vi "_Read Lens Property Settings.vi"() -> (1 "Switches":T1, 2 "Unit":bool, 3 "Spectrum File Path:":path)   [LabVIEW 2015]
uses:
  Type/_Opion Switches.ctl
  <vilib>/Utility/config.llb/Read Key (Path).vi
  <vilib>/Utility/config.llb/Read Key (Boolean).vi
  <vilib>/Utility/config.llb/NI_LVConfig.lvlib
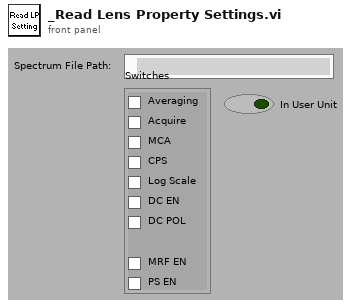
[diagram p1: front panel]
types:
  T1 = typedef "_Opion Switches.ctl" = cluster{"Averaging":bool, "Acquire":bool, "MCA":bool, "CPS":bool, "Log Scale":bool, "DC EN":bool, "DC POL":bool, "MRF EN":bool, "PS EN":bool}
  T2 = typedef "NI_LVConfig.lvlib/Config Data RefNum.ctl" = refnum<k1>
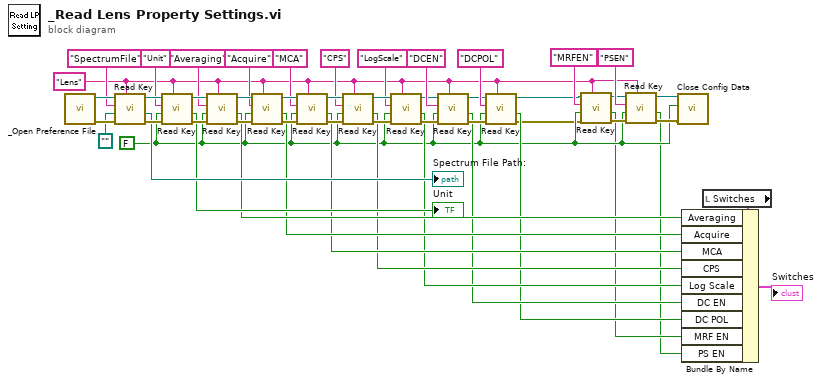
[diagram p0: block diagram]
diagram:
  w5 = FALSE
  w9 = "Lens" ("section")
  n1 = call "_Open Preference File.vi"() -> ("error"=w37:errorcluster, "refnum"=w51:T2)  [unwired: 3 in, 3 out]
  n2 = call-poly <vilib>:"Read Key.vi"("section"=w9, "error in (no error)"=w37, "default value"=path "", "key"="SpectrumFile" ("section"), "refnum"=w51) -> ("error out"=w49:errorcluster, "value"=→"Spectrum File Path:":path, "refnum out"=w48:T2)  [unwired: 4 out]
  n3 = call-poly <vilib>:"Read Key.vi"("section"=w9, "error in (no error)"=w49, "default value"=w5, "key"="Unit" ("section"), "refnum"=w48) -> ("error out"=w47:errorcluster, "value"=→"Unit":bool, "refnum out"=w46:T2)  [unwired: 4 out]
  n4 = call-poly <vilib>:"Read Key.vi"("section"=w9, "error in (no error)"=w47, "default value"=w5, "key"="Averaging" ("section"), "refnum"=w46) -> ("error out"=w45:errorcluster, "value"=w19:bool, "refnum out"=w44:T2)  [unwired: 4 out]
  n5 = call-poly <vilib>:"Read Key.vi"("section"=w9, "error in (no error)"=w45, "default value"=w5, "key"="Acquire" ("section"), "refnum"=w44) -> ("error out"=w43:errorcluster, "value"=w18:bool, "refnum out"=w42:T2)  [unwired: 4 out]
  n6 = call-poly <vilib>:"Read Key.vi"("section"=w9, "error in (no error)"=w43, "default value"=w5, "key"="MCA" ("section"), "refnum"=w42) -> ("error out"=w34:errorcluster, "value"=w17:bool, "refnum out"=w33:T2)  [unwired: 4 out]
  n7 = call-poly <vilib>:"Read Key.vi"("section"=w9, "error in (no error)"=w34, "default value"=w5, "key"="CPS" ("section"), "refnum"=w33) -> ("error out"=w31:errorcluster, "value"=w16:bool, "refnum out"=w30:T2)  [unwired: 4 out]
  n8 = call-poly <vilib>:"Read Key.vi"("section"=w9, "error in (no error)"=w31, "default value"=w5, "key"="LogScale" ("section"), "refnum"=w30) -> ("error out"=w25:errorcluster, "value"=w15:bool, "refnum out"=w24:T2)  [unwired: 4 out]
  n9 = call-poly <vilib>:"Read Key.vi"("section"=w9, "error in (no error)"=w25, "default value"=w5, "key"="DCEN" ("section"), "refnum"=w24) -> ("error out"=w23:errorcluster, "value"=w14:bool, "refnum out"=w27:T2)  [unwired: 4 out]
  n10 = call-poly <vilib>:"Read Key.vi"("section"=w9, "error in (no error)"=w23, "default value"=w5, "key"="DCPOL" ("section"), "refnum"=w27) -> ("error out"=w1:errorcluster, "value"=w13:bool, "refnum out"=w2:T2)  [unwired: 4 out]
  n11 = call-poly <vilib>:"Read Key.vi"("section"=w9, "error in (no error)"=w1, "default value"=w5, "key"="MRFEN" ("section"), "refnum"=w2) -> ("error out"=w8:errorcluster, "value"=w4:bool, "refnum out"=w11:T2)  [unwired: 4 out]
  n12 = call-poly <vilib>:"Read Key.vi"("section"=w9, "error in (no error)"=w8, "default value"=w5, "key"="PSEN" ("section"), "refnum"=w11) -> ("error out"=w7:errorcluster, "value"=w3:bool, "refnum out"=w6:T2)  [unwired: 4 out]
  n13 = call <vilib>:"Close Config Data.vi"("error in (no error)"=w7, "write file if changed (T)"=w5, "refnum"=w6) -> ()  [unwired: 9 out]
  n14 = local read "Switches"() -> (w22:T1)
  n15 = Bundle By Name(cluster=w22, "Averaging"=w19, "Acquire"=w18, "MCA"=w17, "CPS"=w16, "Log Scale"=w15, "DC EN"=w14, "DC POL"=w13, "MRF EN"=w4, "PS EN"=w3) -> (→"Switches":T1)
